vi "adm_test_v1.vi"() -> ()   [LabVIEW 2014]
uses:
  <vilib>/eio/EIONode/EIONode.xnode
  <vilib>/rvi/eio/common/nirviEmuTemplateMethod_errors.vi
panel:
  out "mt_p2":u32
  out "Dp1_d (T)":fxp<+/-,64,58>
  out "omega_p1 (T)":fxp<+/-,36,13>
  out "mt_p1":u32
  out "rad_p2":fxp<+/-,64,63>
  out "rad_p1":fxp<+/-,48,33>
  out "D_p2":fxp<+/-,64,104>
  out "F_mot2mag":fxp<+/-,64,32>
  in  "Mag. factor_p":fxp<+/-,32,1>
  out "Encoder Position_p2":i32
  out "D_p1":fxp<+/-,64,72>
  in  "Belt_out_p":fxp<+/-,40,-10>
  in  "Belt_in_p":fxp<+/-,20,-5>
  out "Encoder Position_p1":i32
  in  "Encoder Reset_p":bool
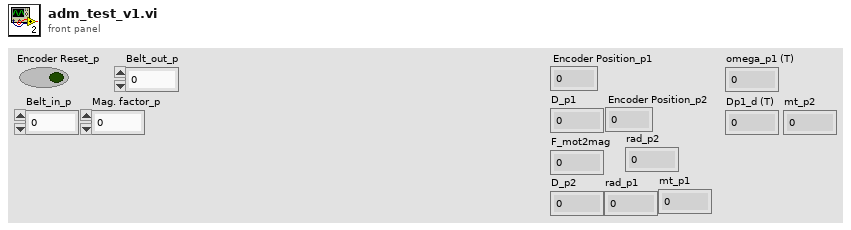
[diagram p1: front panel]
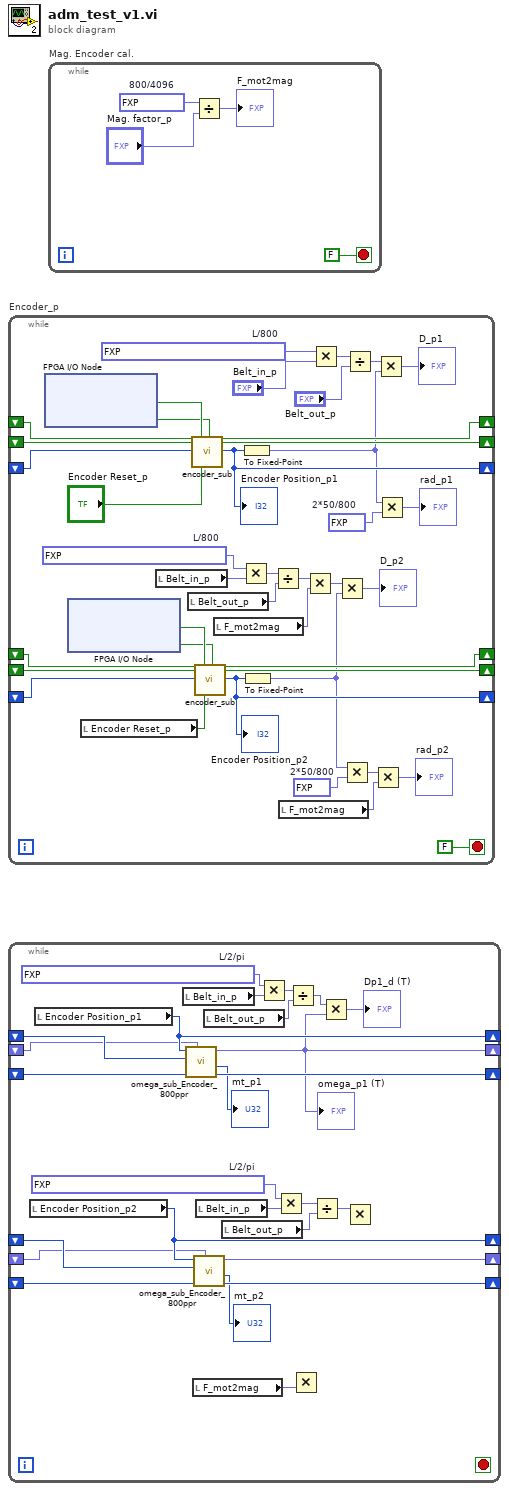
[diagram p0: block diagram]
diagram:
  n1 = while "Encoder_p" {
    shift-right: [w38] -> _
    shift-left: _ -> [w39]
    shift-right: [w37] -> _
    shift-left: _ -> [w36]
    shift-right: [w33] -> _
    shift-left: _ -> [w35]
    shift-right: [w22] -> _
    shift-left: _ -> [w21]
    shift-right: [w23] -> _
    shift-left: _ -> [w20]
    shift-right: [w18] -> _
    shift-left: _ -> [w19]
    stop <- FALSE stop-if-true
    w6 = fxp<+/-,16,1> 0.125  # 2*50/800
    w8 = fxp<+/-,16,1> 0.125  # 2*50/800
    w13 = fxp<+/-,20,-5> 0.002499997615814209  # L/800
    w31 = fxp<+/-,20,-5> 0.002499997615814209  # L/800
    n2 = xnode "FPGA I/O Node"() -> ("Mod7/DIO0"=w41:bool, "Mod7/DIO1"=w40:bool)  [unwired: 2 in, 2 out]
    n3 = xnode "FPGA I/O Node"() -> ("Mod7/DIO4"=w25:bool, "Mod7/DIO5"=w24:bool)  [unwired: 2 in, 2 out]
    n4 = local read "Encoder Reset_p"() -> (w26:bool)
    n5 = local read "Belt_in_p"() -> (w15:fxp<+/-,20,-5>)
    n6 = local read "Belt_out_p"() -> (w14:fxp<+/-,40,-10>)
    n7 = call "encoder_sub.vi"("A_pre"=w39, "B_pre"=w36, "Encoder Position_pre"=w35, "A input"=w41, "Encoder Position Reset"="Encoder Reset_p", "B input"=w40) -> ("A"=w38:bool, "B"=w37:bool, "Encoder Position (Counts)"=w33:i32)  [unwired: 19 in]
    "Encoder Position_p1" <- w33
    n8 = call "encoder_sub.vi"("A_pre"=w21, "B_pre"=w20, "Encoder Position_pre"=w19, "A input"=w25, "Encoder Position Reset"=w26, "B input"=w24) -> ("A"=w22:bool, "B"=w23:bool, "Encoder Position (Counts)"=w18:i32)  [unwired: 19 in]
    "Encoder Position_p2" <- w18
    n9 = local read "F_mot2mag"() -> (w12:fxp<+/-,64,32>)
    n10 = Multiply(x=w13, y=w15) -> (x*y=w17:fxp<+/-,40,-10>)
    n11 = To Fixed-Point(number=w33) -> (fixed-point=w9:fxp<+/-,32,32>)  [unwired: 1 in]
    n12 = To Fixed-Point(number=w18) -> (fixed-point=w3:fxp<+/-,32,32>)  [unwired: 1 in]
    n13 = Divide(x=w17, y=w14) -> (x/y=w16:fxp<+/-,64,40>)
    n14 = local read "F_mot2mag"() -> (w4:fxp<+/-,64,32>)
    n15 = Multiply(x=w16, y=w12) -> (x*y=w11:fxp<+/-,64,72>)
    n16 = Multiply(x=w31, y="Belt_in_p") -> (x*y=w32:fxp<+/-,40,-10>)
    n17 = Multiply(x=w11, y=w3) -> (x*y=→"D_p2":fxp<+/-,64,104>)
    n18 = Multiply(x=w3, y=w6) -> (x*y=w5:fxp<+/-,48,33>)
    n19 = Divide(x=w32, y="Belt_out_p") -> (x/y=w28:fxp<+/-,64,40>)
    n20 = Multiply(x=w5, y=w4) -> (x*y=→"rad_p2":fxp<+/-,64,63>)
    n21 = Multiply(x=w28, y=w9) -> (x*y=→"D_p1":fxp<+/-,64,72>)
    n22 = Multiply(x=w9, y=w8) -> (x*y=→"rad_p1":fxp<+/-,48,33>)
  }
  n23 = while {
    shift-right: [w66] -> _
    shift-left: _ -> [w67]
    shift-right: [w56] -> _
    shift-left: _ -> [w65]
    shift-right: [w64] -> _
    shift-left: _ -> [w63]
    shift-right: [w52] -> _
    shift-left: _ -> [w51]
    shift-right: [w53] -> _
    shift-left: _ -> [w50]
    shift-right: [w54] -> _
    shift-left: _ -> [w49]
    stop <- _ stop-if-true
    w47 = fxp<+/-,32,0> 0.3183098859153688  # L/2/pi
    w61 = fxp<+/-,32,0> 0.3183098859153688  # L/2/pi
    n24 = local read "Encoder Position_p2"() -> (w52:i32)
    n25 = local read "Encoder Position_p1"() -> (w66:i32)
    n26 = local read "Belt_in_p"() -> (w60:fxp<+/-,20,-5>)
    n27 = call "omega_sub_Encoder_800ppr.vi"("omega_pre"=w65, "ticks_m_pre"=w63, "count_pre"=w67, "count"=w66) -> ("ticks_m"=w64:u32, "mt"=→"mt_p1":u32, "omega"=w56:fxp<+/-,36,13>)  [unwired: 5 in]
    "omega_p1 (T)" <- w56
    n28 = local read "F_mot2mag"() -> (w43:fxp<+/-,64,32>)
    n29 = call "omega_sub_Encoder_800ppr.vi"("omega_pre"=w50, "ticks_m_pre"=w49, "count_pre"=w51, "count"=w52) -> ("ticks_m"=w54:u32, "mt"=→"mt_p2":u32, "omega"=w53:fxp<+/-,36,13>)  [unwired: 5 in]
    n30 = local read "Belt_in_p"() -> (w48:fxp<+/-,20,-5>)
    n31 = local read "Belt_out_p"() -> (w58:fxp<+/-,40,-10>)
    n32 = local read "Belt_out_p"() -> (w45:fxp<+/-,40,-10>)
    n33 = Multiply(x=w61, y=w60) -> (x*y=w59:fxp<+/-,52,-5>)
    n34 = Multiply(x=w47, y=w48) -> (x*y=w46:fxp<+/-,52,-5>)
    n35 = Divide(x=w59, y=w58) -> (x/y=w57:fxp<+/-,64,45>)
    n36 = Multiply(y=w43) -> ()  [unwired: 1 in, 1 out]
    n37 = Divide(x=w46, y=w45) -> (x/y=w44:fxp<+/-,64,45>)
    n38 = Multiply(x=w57, y=w56) -> (x*y=→"Dp1_d (T)":fxp<+/-,64,58>)
    n39 = Multiply(x=w44) -> ()  [unwired: 1 in, 1 out]
  }
  n40 = while "Mag. Encoder cal." {
    stop <- FALSE stop-if-true
    w71 = fxp<+,32,0> 0.1953125  # 800/4096
    n41 = Divide(x=w71, y="Mag. factor_p") -> (x/y=→"F_mot2mag":fxp<+/-,64,32>)
  }
